vi "Initial Path Plot Sub_VI.vi"(10 "Motion Inputs":T3) -> (1 "Accel Array":dbl[](graph), 2 "Velocity Array":dbl[](graph), 3 "Displacement Array":dbl[](graph), 7 "Motion Outputs":T2)   [LabVIEW 2017]
panel:
  out "Motion Planning Outputs":T1
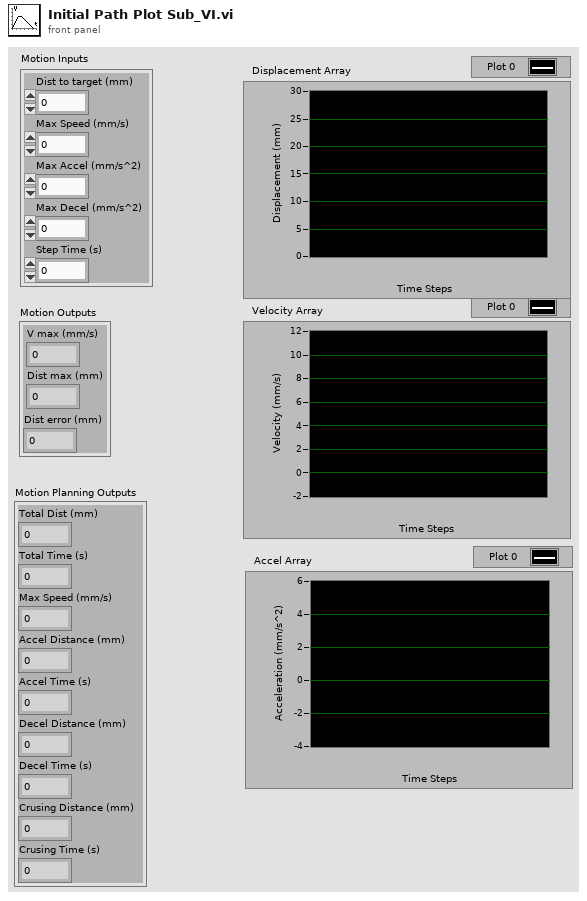
[diagram p1: front panel]
types:
  T1 = cluster{"Crusing Time (s)":dbl, "Decel Time (s)":dbl, "Accel Time (s)":dbl, "Total Time (s)":dbl, "Accel Distance (mm)":dbl, "Decel Distance (mm)":dbl, "Crusing Distance (mm)":dbl, "Total Dist (mm)":dbl, "Max Speed (mm/s)":dbl}
  T2 = cluster{"V max (mm/s)":dbl, "Dist max (mm)":dbl, "Dist error (mm)":dbl}
  T3 = cluster{"Dist to target (mm)":dbl, "Max Speed (mm/s)":dbl, "Max Accel (mm/s^2)":dbl, "Max Decel (mm/s^2)":dbl, "Step Time (s)":dbl}
  T4 = cluster{"Decel Time (s)":dbl, "Accel Time (s)":dbl, "Total Time (s)":dbl, "Accel (mm/s^2)":dbl, "Decel (mm/s^2)":dbl, "Time step (s)":dbl}
  T5 = cluster{" Distance target (mm)":dbl, "Max Accel (mm/s^2)":dbl, "Max Decel (mm/s^2)":dbl, "Velocity Limit (mm/s) ":dbl}
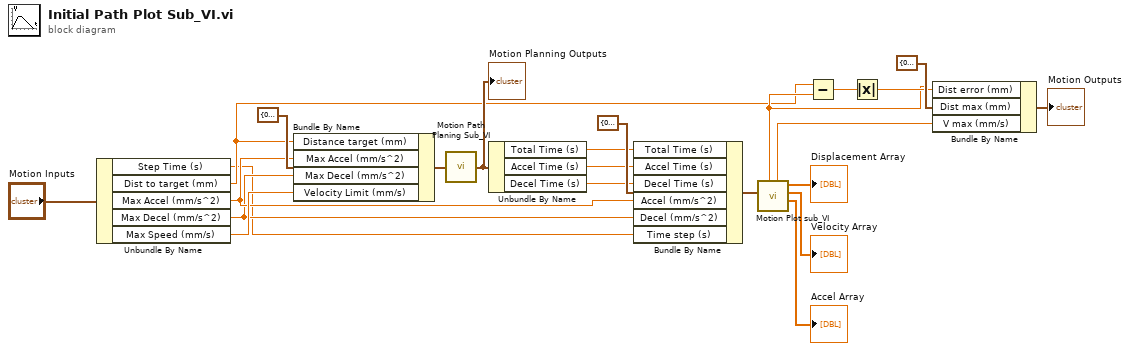
[diagram p0: block diagram]
diagram:
  n1 = Unbundle By Name("Motion Inputs") -> ("Step Time (s)"=w1:dbl, "Dist to target (mm)"=w8:dbl, "Max Accel (mm/s^2)"=w3:dbl, "Max Decel (mm/s^2)"=w2:dbl, "Max Speed (mm/s)"=w19:dbl)
  n2 = Bundle By Name(cluster=T5 {" Distance target (mm)"=0.0, "Max Accel (mm/s^2)"=0.0, "Max Decel (mm/s^2)"=0.0, "Velocity Limit (mm/s) "=0.0} ("Motion Planning Inputs"), "Distance target (mm)"=w8, "Max Accel (mm/s^2)"=w3, "Max Decel (mm/s^2)"=w2, "Velocity Limit (mm/s)"=w19) -> (w17:T5)
  n3 = call "Motion Path Planing Sub_VI.vi"("Motion Planning Inputs"=w17) -> ("Motion Planning Outputs"=w15:T1)  [unwired: 5 in, 1 out]
  "Motion Planning Outputs" <- w15
  n4 = Unbundle By Name(w15) -> ("Total Time (s)"=w6:dbl, "Accel Time (s)"=w5:dbl, "Decel Time (s)"=w4:dbl)
  n5 = Bundle By Name(cluster=T4 {"Decel Time (s)"=0.0, "Accel Time (s)"=0.0, "Total Time (s)"=0.0, "Accel (mm/s^2)"=0.0, "Decel (mm/s^2)"=0.0, "Time step (s)"=0.01} ("Motion Parameters"), "Total Time (s)"=w6, "Accel Time (s)"=w5, "Decel Time (s)"=w4, "Accel (mm/s^2)"=w3, "Decel (mm/s^2)"=w2, "Time step (s)"=w1) -> (w13:T4)
  n6 = call "Motion Plot sub_VI.vi"("Motion Parameters"=w13) -> ("Acceleration"=→"Accel Array":dbl[], "Velocity"=→"Velocity Array":dbl[], "Displacement"=→"Displacement Array":dbl[], "V max (mm/s)"=w7:dbl, "Dist max (mm)"=w9:dbl)  [unwired: 4 in]
  n7 = Subtract(x=w8, y=w9) -> (x-y=w22:dbl)
  n8 = Absolute Value(x=w22) -> (abs(x)=w18:dbl)
  n9 = Bundle By Name(cluster=T2 {"V max (mm/s)"=0.0, "Dist max (mm)"=0.0, "Dist error (mm)"=0.0} ("Motion Outputs 2"), "Dist error (mm)"=w18, "Dist max (mm)"=w9, "V max (mm/s)"=w7) -> (→"Motion Outputs":T2)
